vi "Active Noise Control (RT).vi"() -> ()   [LabVIEW 2023]
doc: "This VI runs on an RT target. This VI downloads the Active Noise Control (FPGA) VI to FPGA, runs the Active Noise Control (FPGA) VI on FPGA, communicates with the Active Noise Control (FPGA) VI to read and display the primary noise, control waveform, and the noise at the location of interest. \n\nComplete the following steps to use this example.\n\n1. Configure the settings for secondary path modeling in the <b>Secondary Paht Modeling</b> page.\n\n2. Configure the settings for active noise control in the <b>Active Noise Control</b> page.\n \n3. Run this VI. This VI then switches to the <b>Secondary Path Modeling</b> page. When the secondary path modeling is complete, this VI switches to the <b>Active Noise Control</b> page.\n\n4. Click the <b>Control</b> button. Verify whether the noise is reduced."
uses:
  <vilib>/rvi/interface/nirviOpenFPGA/nirviOpenFPGA.xnode
  <vilib>/rvi/interface/nirviReadWriteControl/nirviReadWriteControl.xnode
  <vilib>/rvi/interface/nirviCloseFPGA/nirviCloseFPGA.xnode
  <vilib>/rvi/interface/nirviMethod/nirviMethod.xnode
  FPGA Bitfiles/activenoisecontr_FPGATarget_ActiveNoiseContr_QJDRzKuGyKY.lvbitx
  Active Noise Control (FPGA).vi
  <vilib>/rvi/errors/niLvFpgaMergeErrorWithErrorCode.vi
  <vilib>/userdefined/High Color/nirio_resource_hc.ctl
panel:
  in  "Tab Control":T1(tab)
  in  "Gain for d(n)":i32=2
  in  "RIO Device":T2="RIO0"
  in  "Step Size (LMS)":fxp<+/-,16,-5>=0.0009999275207519531 format="%#.3g"
  in  "Modeling Time (s)":i32=5
  out "x(n)":dbl[](graph)
  out "d(n)":dbl[](graph)
  out "e(n)":dbl[](graph)
  in  "Step Size (FXLMS)":fxp<+/-,16,-2>=0.049999237060546875 format="%#.3g"
  in  "Control":bool
  in  "Reset":bool
  out "Secondary Path":dbl[](graph)
  out "Noise level":dbl[](graph)
  in  "Noise Frequency (Hz)":fxp<+/-,16,16>=120.0
  in  "Stop":bool
  out "Signals":dbl[](graph)
  # "Refer to the Active Noise Control topic in the LabVIEW Help for more information about the background of active noise control. Select Help>>Show Context Help and move the cursor over the VI icon of this example for more information."
  # "Secondary Path Modeling"
  # "Active Noise Control"
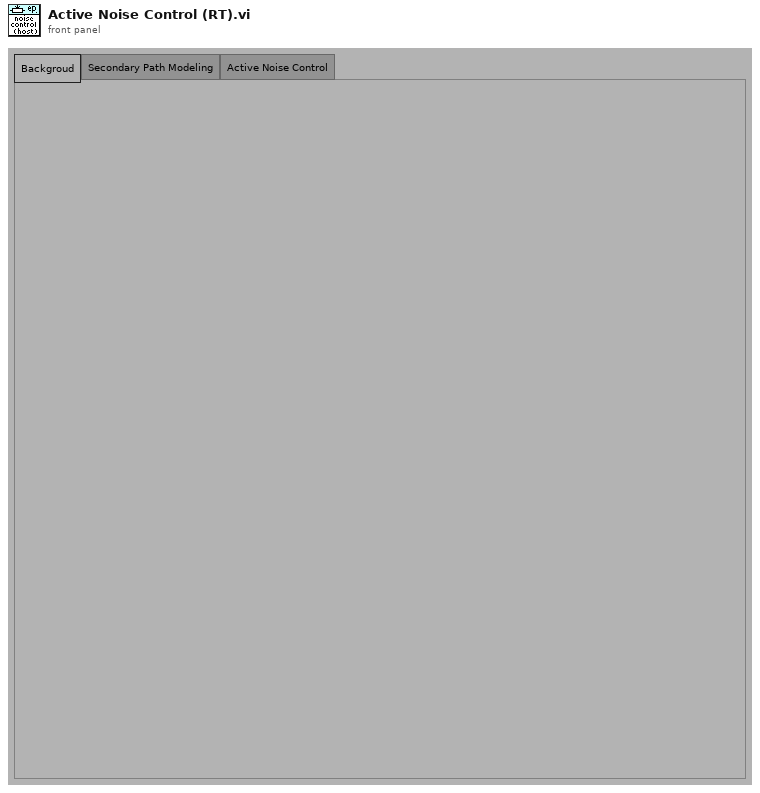
[diagram p1: front panel]
types:
  T1 = enum32{"Backgroud", "Secondary Path Modeling", "Active Noise Control"}
  T2 = typedef "nirio_resource_hc.ctl" = tag
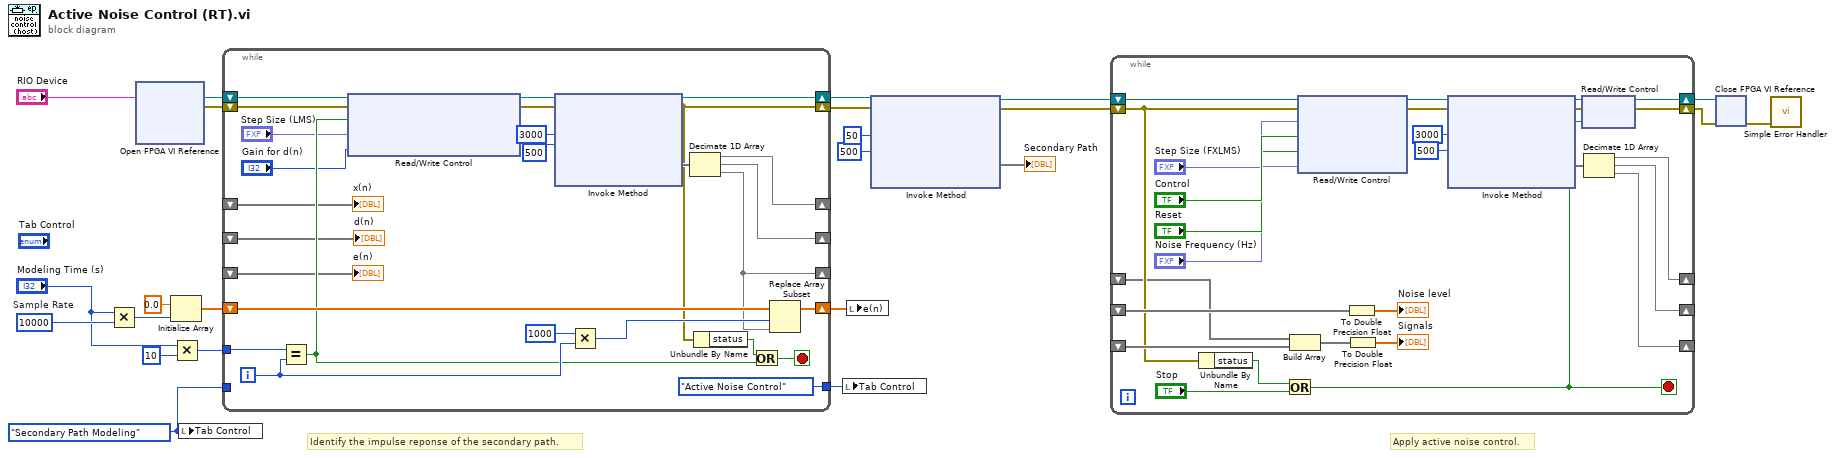
[diagram p0: block diagram]
diagram:
  w2 = T1."Secondary Path Modeling" ("Tab Control")
  w13 = 10000  # Sample Rate
  # "Apply active noise control."
  # "Identify the impulse reponse of the secondary path."
  n1 = Multiply(x="Modeling Time (s)", y=w13) -> (x*y=w12:i32)
  n2 = xnode "Open FPGA VI Reference"("resource name"="RIO Device") -> ("FPGA VI Reference Out"=w23:refnum<k20>, "error out"=w8:errorcluster)  [unwired: 1 in]
  n3 = Initialize Array(0.0 ("element"), w12) -> (w17:dbl[])
  n4 = Multiply(x="Modeling Time (s)", y=10) -> (x*y=w9:i32)
  n5 = local write "Tab Control"(w2) -> ()
  n6 = while {
    shift-right: [w43] -> w1
    shift-left: w17 -> [w44]
    shift-right: [w36] -> _
    shift-left: _ -> [w34]
    shift-right: [w35] -> _
    shift-left: _ -> [w33]
    tunnel: w9 -> [w32]
    shift-right: [w28] -> w7
    shift-left: w8 -> [w31]
    tunnel: [T1."Active Noise Control" ("Tab Control")] -> w3
    tunnel: w2 -> [_]
    shift-right: [w25] -> _
    shift-left: _ -> [w24]
    shift-right: [w48] -> w22
    shift-left: w23 -> [w50]
    i -> [w41]
    stop <- w29 stop-if-true
    n7 = Equal?(x=w32, y=w41) -> (x = y?=w40:bool)
    n8 = xnode "Read/Write Control"("FPGA VI Reference In"=w50, "error in"=w31, "stop modeling"=w40, "step size (LMS)"="Step Size (LMS)", "gain for microphone channel"="Gain for d(n)") -> ("FPGA VI Reference Out"=w49:refnum<k20>, "error out"=w30:errorcluster)
    n9 = xnode "Invoke Method"("FPGA VI Reference In"=w49, "error in"=w30, "Number of Elements"=u32 3000, "Timeout (ms)"=500) -> ("FPGA VI Reference Out"=w48:refnum<k20>, "error out"=w28:errorcluster, "Data"=w46:void[])  [unwired: 1 out]
    n10 = Multiply(x=1000 ("y"), y=w41) -> (x*y=w45:i32)
    n11 = Decimate 1D Array(w46) -> (w36:void[], w35:void[], w25:void[])
    n12 = Unbundle By Name(w28) -> ("status"=w27:bool)
    n13 = Or(x=w27, y=w40) -> (x .or. y?=w29:bool)
    n14 = Replace Array Subset(array=w44, new element=w25, index=w45) -> (w43:dbl[])
    "x(n)" <- w34
    "d(n)" <- w33
    "e(n)" <- w24
  }
  n15 = local write "Tab Control"(w3) -> ()
  n16 = local write "e(n)"(w1) -> ()
  n17 = xnode "Invoke Method"("FPGA VI Reference In"=w22, "error in"=w7, "Number of Elements"=u32 50, "Timeout (ms)"=500) -> ("FPGA VI Reference Out"=w16:refnum<k20>, "error out"=w6:errorcluster, "Data"=→"Secondary Path":void[])  [unwired: 1 out]
  n18 = while {
    shift-right: [w67] -> _
    shift-left: _ -> [w58]
    shift-right: [w66] -> _
    shift-left: _ -> [w64]
    shift-right: [w65] -> _
    shift-left: _ -> [w63]
    shift-right: [w52] -> w5
    shift-left: w6 -> [w61]
    shift-right: [w53] -> w15
    shift-left: w16 -> [w77]
    stop <- w51 stop-if-true
    n19 = Unbundle By Name(w61) -> ("status"=w60:bool)
    n20 = Or(x=w60, y="Stop") -> (x .or. y?=w51:bool)
    n21 = Build Array(w58, w63) -> (w59:void[])
    n22 = xnode "Read/Write Control"("FPGA VI Reference In"=w77, "error in"=w61, "step size (FXLMS)"="Step Size (FXLMS)", "control on"="Control", "reset"="Reset", "frequency (Hz)"="Noise Frequency (Hz)") -> ("FPGA VI Reference Out"=w76:refnum<k20>, "error out"=w62:errorcluster)
    n23 = To Double Precision Float(number=w64) -> (double precision float=→"Noise level":dbl[])
    n24 = To Double Precision Float(number=w59) -> (double precision float=→"Signals":dbl[])
    n25 = xnode "Invoke Method"("FPGA VI Reference In"=w76, "error in"=w62, "Number of Elements"=u32 3000, "Timeout (ms)"=500) -> ("FPGA VI Reference Out"=w55:refnum<k20>, "error out"=w54:errorcluster, "Data"=w74:void[])  [unwired: 1 out]
    n26 = xnode "Read/Write Control"("FPGA VI Reference In"=w55, "error in"=w54, "stop"=w51) -> ("FPGA VI Reference Out"=w53:refnum<k20>, "error out"=w52:errorcluster)
    n27 = Decimate 1D Array(w74) -> (w67:void[], w66:void[], w65:void[])
  }
  n28 = xnode "Close FPGA VI Reference"("FPGA VI Reference In"=w15, "error in"=w5) -> ("error out"=w4:errorcluster)
  n29 = call <vilib>:"Simple Error Handler.vi"("error in (no error)"=w4) -> ()  [unwired: 1 in, 8 out]
